vi "calc_gigaseal_slope.vi"(10 "num samples":i32, 11 "gigasealing array":dbl[](array[numeric])) -> (3 "slope (Mohm / s)":dbl)   [LabVIEW 2015]
uses:
  <vilib>/Analysis/NI_AALPro.lvlib
  <vilib>/Analysis/6fits.llb/Curve Fitting Criteria.ctl
panel:
  out "Array":dbl[](array[numeric])
  out "last x elements":dbl[](array[numeric])
  # "calculate gigasealing slope"
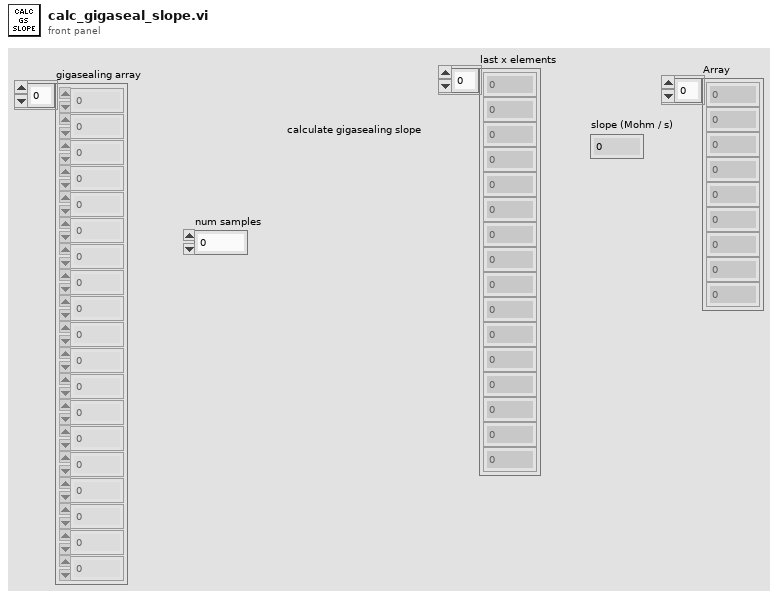
[diagram p1: front panel]
types:
  T1 = typedef "NI_AALPro.lvlib/Curve Fitting Criteria.ctl" = u16
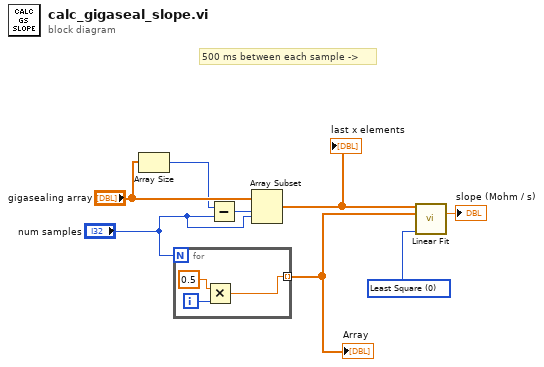
[diagram p0: block diagram]
diagram:
  w4 = T1 0 items=["Least Square", "Least Absolute Residual", "Bisquare"] ("method")
  # "500 ms between each sample ->"
  n1 = Array Size(array="gigasealing array") -> (size(s)=w7:i32)
  n2 = for {
    N: "num samples" -> [_]
    tunnel: [w9] -> w1 mode=indexing
    i -> [w11]
    n3 = Multiply(x=0.5, y=w11) -> (x*y=w9:dbl)
  }
  "Array" <- w1
  n4 = Subtract(x=w7, y="num samples") -> (x-y=w6:i32)
  n5 = Array Subset(array="gigasealing array", index=w6, length="num samples") -> (w5:dbl[])
  "last x elements" <- w5
  n6 = call <vilib>:"Linear Fit.vi"("Y"=w5, "X"=w1, "method"=w4) -> ("slope"=→"slope (Mohm / s)":dbl)  [unwired: 8 in, 4 out]
